vi "Application Launcher.vi"(8 "error in (no error)":errorcluster, 9 "Toggle?":bool, 11 "VI reference":refnum<vi>) -> (0 "error out":errorcluster, 3 "VI reference out":refnum<vi>)   [LabVIEW 2012]
doc: "Takes a VI reference and checks its state; if it is already running, it brings its front panel to the front of the screen. If it isn't running, it launches it."
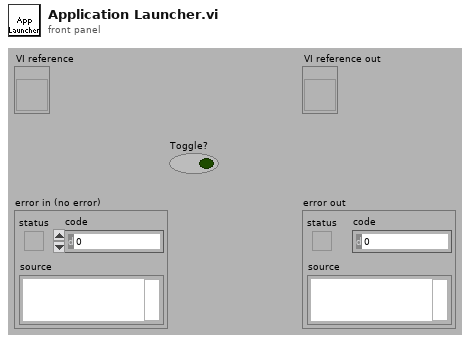
[diagram p1: front panel]
types:
  T1 = enum32{"Bad", "Idle", "Run top level", "Running"}
  T2 = enum32{"Invalid", "Standard", "Closed", "Hidden", "Minimized", "Maximized"}
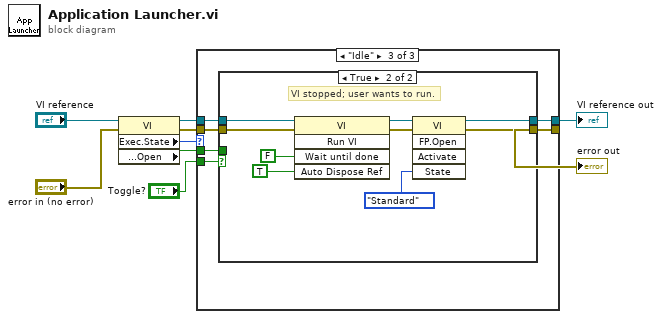
[diagram p0: block diagram]
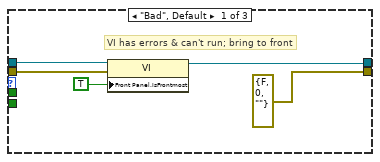
[diagram p2: hidden frame]
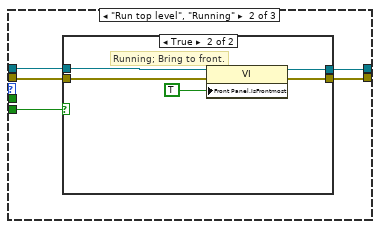
[diagram p3: hidden frame]
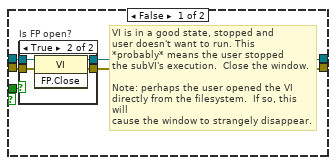
[diagram p5: hidden frame]
diagram:
  n1 = property class="VI"(reference="VI reference", error in="error in (no error)") -> (reference out=w8:refnum<vi>, error out=w9:errorcluster, "Exec.State"=w7:T1, "Front Panel.Open"=w1:bool)
  n2 = case shown="\"Idle\"" w7 {
    tunnel: w9 -> [w13 w18 w31]
    tunnel: w8 -> [w14 w19 w32]
    tunnel: [w11 w17 w30] -> w4
    tunnel: [errorcluster {"status"=FALSE, "code"=0, "source"=""} ("error out") w16 w29] -> w3
    tunnel: "Toggle?" -> [_ w15 w28]
    tunnel: w1 -> [_ _ w27]
    frame "Bad", Default {
      # "VI has errors & can't run; bring to front"
      n3 = property class="VI"(reference=w14, error in=w13, "Front Panel.IsFrontmost"=TRUE ("Front Panel Window:Is Frontmost")) -> (reference out=w11:refnum<vi>)  [unwired: 1 out]
    }
    frame "Run top level", "Running" {
      n4 = case shown="True" w15 {
        tunnel: w19 -> [w20 w26]
        tunnel: w18 -> [w21 w25]
        tunnel: [w20 w24] -> w17
        tunnel: [w21 w23] -> w16
        frame False {
          # "Running; user didn't toggle\nso don't bring to front."
        }
        frame True {
          # "Running; Bring to front."
          n5 = property class="VI"(reference=w26, error in=w25, "Front Panel.IsFrontmost"=TRUE ("Front Panel Window:Is Frontmost")) -> (reference out=w24:refnum<vi>, error out=w23:errorcluster)
        }
      }
    }
    frame "Idle" {
      n6 = case shown="True" w28 {
        tunnel: w32 -> [w37 w52]
        tunnel: w31 -> [w36 w51]
        tunnel: [w35 w46] -> w30
        tunnel: [w34 w45] -> w29
        tunnel: w27 -> [w33 _]
        frame False {
          # "VI is in a good state, stopped and \nuser doesn't want to run. This\n*probably* means the user stopped\nthe subVI's execution.  Close the window.\n\nNote: perhaps the user opened the VI\ndirectly from the filesystem.  If so, this will\ncause the window to strangely disappear."
          n7 = case "Is FP open?" shown="True" w33 {
            tunnel: w37 -> [w39 w43]
            tunnel: w36 -> [w38 w42]
            tunnel: [w39 w41] -> w35
            tunnel: [w38 w40] -> w34
            frame False {
            }
            frame True {
              n8 = invoke class="VI" method="FP.Close"(reference=w43, error in=w42) -> (reference out=w41:refnum<vi>, error out=w40:errorcluster)  [unwired: 1 in, 1 out]
            }
          }
        }
        frame True {
          # "VI stopped; user wants to run."
          n9 = invoke class="VI" method="Run VI"(reference=w52, error in=w51, "Wait until done"=FALSE ("Wait Until Done"), "Auto Dispose Ref"=TRUE ("Auto Dispose Reference")) -> (reference out=w49:refnum<vi>, error out=w48:errorcluster)  [unwired: 1 in, 3 out]
          n10 = invoke class="VI" method="FP.Open"(reference=w49, error in=w48, "State"=T2."Standard") -> (reference out=w46:refnum<vi>, error out=w45:errorcluster)  [unwired: 2 in, 3 out]
        }
      }
    }
  }
  "VI reference out" <- w4
  "error out" <- w3
